vi "Move to New Position.vi"(7 "Curr Filter":i32, 8 "error in (no error)":errorcluster, 9 "Target Filter":i32, 10 "Filter Wheel (0:n-1)":i32, 11 "FW Arduino Control in":refnum<class "FW Arduino Control.lvclass">) -> (0 "error out":errorcluster, 1 "Actual Distance":i32[](array[numeric]), 2 "Log":string, 3 "FW Arduino Control out":refnum<class "FW Arduino Control.lvclass">)   [LabVIEW 2024, in "FW Arduino Control.lvclass"]
uses:
  FW Arduino Control.lvclass
  Filter Wheel Object/Filter Wheel.lvclass
  FW Arduino Control.lvclass/FW Arduino Control.ctl
  <vilib>/Utility/error.llb/Trim Whitespace One-Sided.vi
panel:
  out "notches":i32
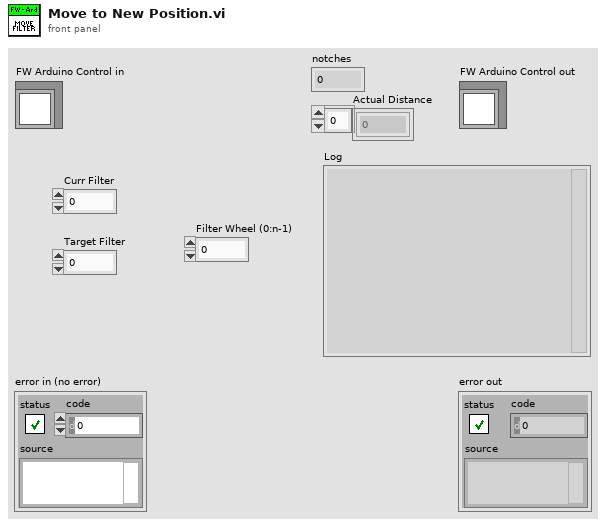
[diagram p1: front panel]
types:
  T1 = typedef "Filter Wheel.lvclass/Filter Wheel configuration.ctl" = cluster{"Num Wheels":i32, "Filters":T2[], "Invalid Combinations":i32[][], "Addr":refnum<visa-resource-name>, "Name":string, "Simulate":bool, "Default Speed":u16, "Homing":T3[]}
  T2 = typedef "Filter Wheel.lvclass/Filter Wheel Details.ctl" = cluster{"Names":string[], "Relative Position":i32[], "Wheel Name":string, "Size":i32}
  T3 = typedef "Filter Wheel Arduino Homing cluster.ctl" = cluster{"Direction (F: CW)":bool, "Speed":i32, "Accel":i32, "Error Cnts":i32, "Homing Delta":i32}
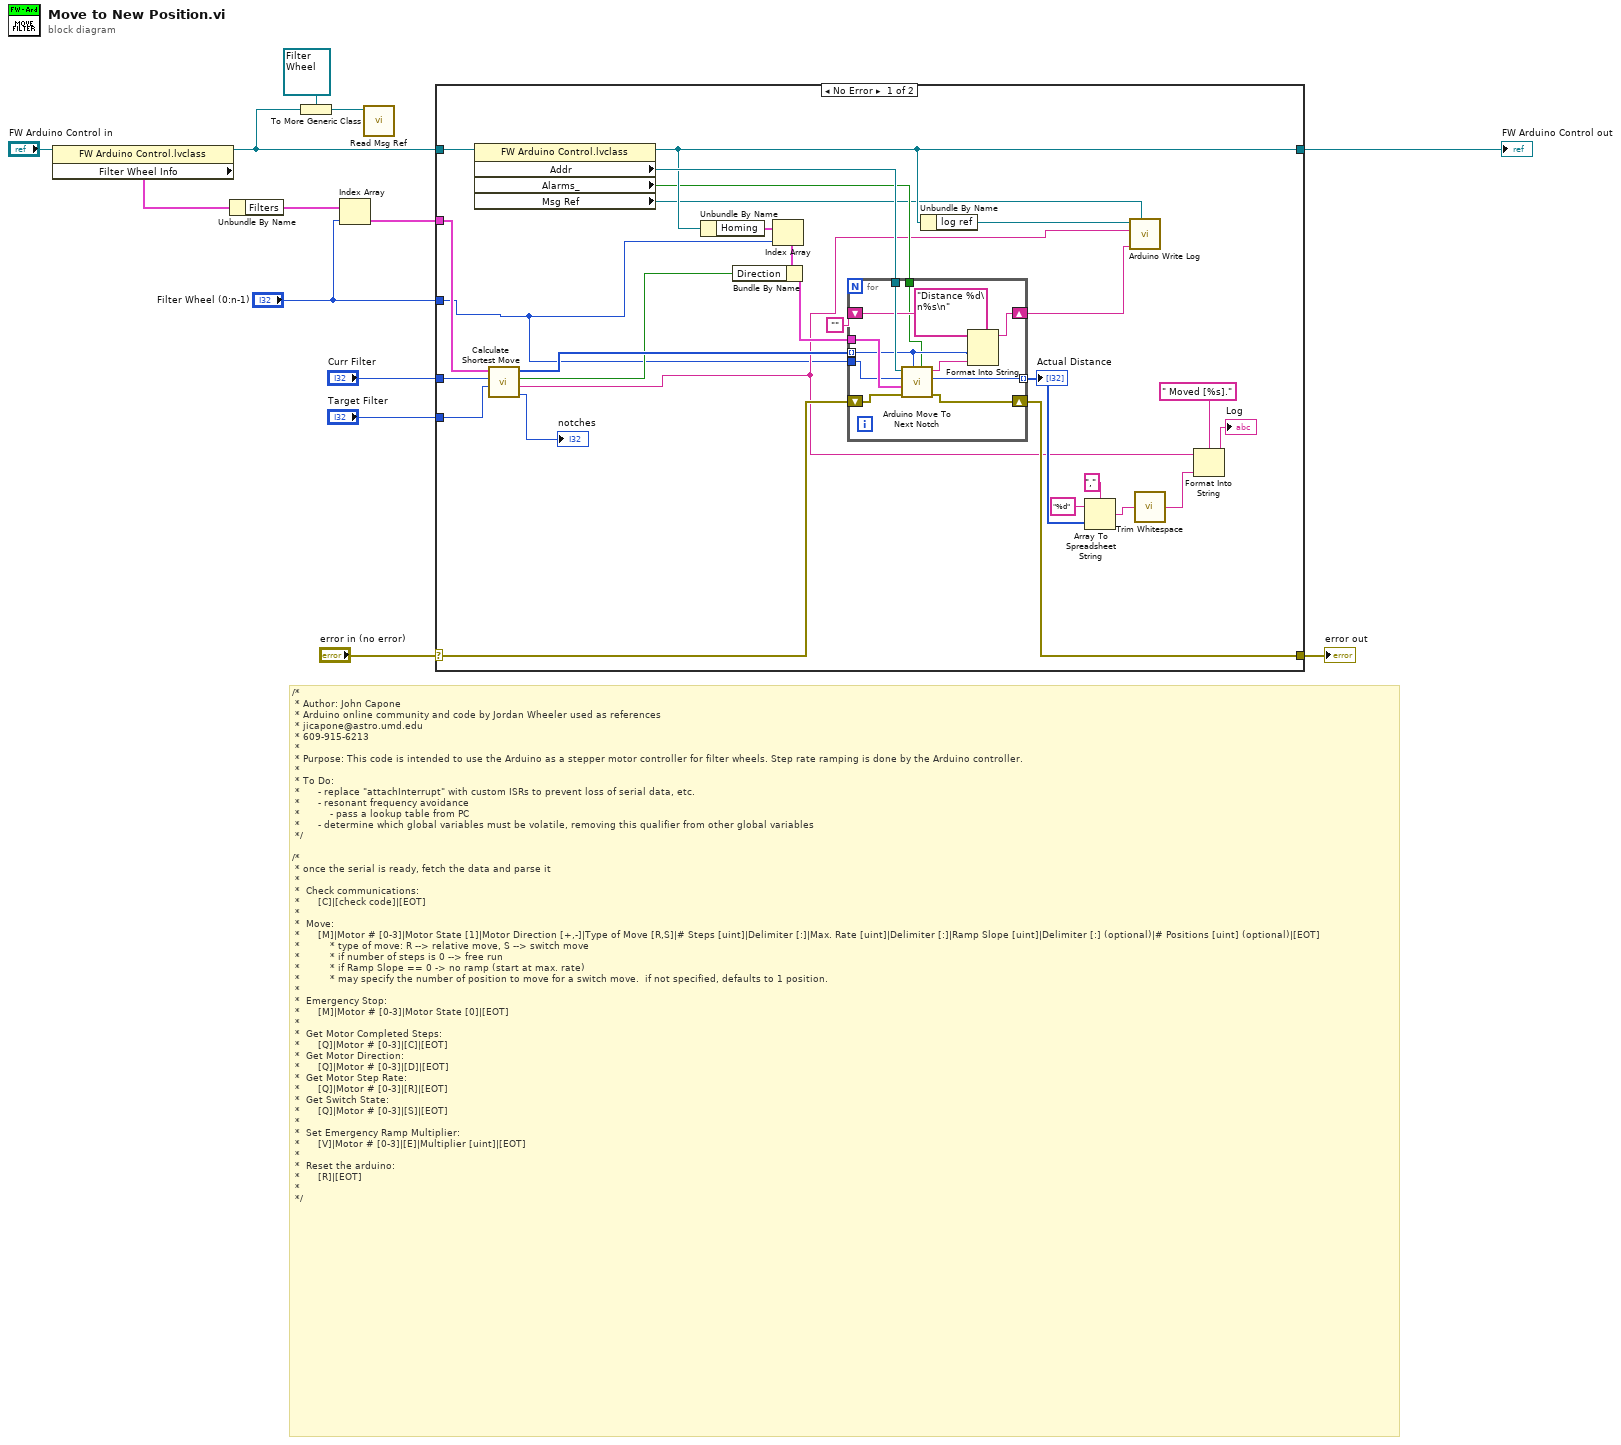
[diagram p0: block diagram]
diagram:
  # "/*\n * Author: John Capone\n * Arduino online community and code by Jordan Wheeler used as references\n * jicapone@astro.umd.edu\n * 609-915-6213\n * \n * Purpose: This code is intended to use the Arduino as a stepper motor controller for filter wheels. Step rate ramping is done by the Arduino controller.\n * \n * To Do:\n *      - replace \"attachInterrupt\" with custom ISRs to prevent loss of serial data, etc.\n *      - resonant frequency avoidance\n *          - pass a lookup table from PC\n *      - determine which global variables must be volatile, removing this qualifier from other global variables\n */\n\n/* \n * once the serial is ready, fetch the data and parse it\n *\n *  Check communications:\n *      [C]|[check code]|[EOT]\n *\n *  Move:\n *      [M]|Motor # [0-3]|Motor State [1]|Motor Direction [+,-]|Type of Move [R,S]|# Steps [uint]|Delimiter [:]|Max. Rate [uint]|Delimiter [:]|Ramp Slope [uint]|Delimiter [:] (optional)|# Positions [uint] (optional)|[EOT]\n *          * type of move: R --> relative move, S --> switch move\n *          * if number of steps is 0 --> free run\n *          * if Ramp Slope == 0 -> no ramp (start at max. rate)\n *          * may specify the number of position to move for a switch move.  if not specified, defaults to 1 position.\n *\n *  Emergency Stop:\n *      [M]|Motor # [0-3]|Motor State [0]|[EOT]\n *\n *  Get Motor Completed Steps:\n *      [Q]|Motor # [0-3]|[C]|[EOT]\n *  Get Motor Direction:\n *      [Q]|Motor # [0-3]|[D]|[EOT]\n *  Get Motor Step Rate:\n *      [Q]|Motor # [0-3]|[R]|[EOT]\n *  Get Switch State:\n *      [Q]|Motor # [0-3]|[S]|[EOT]\n *\n *  Set Emergency Ramp Multiplier:\n *      [V]|Motor # [0-3]|[E]|Multiplier [uint]|[EOT]\n *\n *  Reset the arduino:\n *      [R]|[EOT]\n *\n */"
  n1 = property class="FW Arduino Control.lvclass"(reference="FW Arduino Control in") -> (reference out=w1:refnum<class "FW Arduino Control.lvclass">, "Filter Wheel Info"=w7:T1)  [unwired: 1 in, 1 out]
  n2 = Unbundle By Name(w7) -> ("Filters"=w6:T2[])
  n3 = To More Generic Class(target class=refnum<class "Filter Wheel.lvclass"> refnum ("Filter Wheel.lvclass"), reference=w1) -> (generic class reference=w2:refnum<class "Filter Wheel.lvclass">)
  n4 = Index Array(array=w6, index="Filter Wheel (0:n-1)") -> (element=w4:T2)
  n5 = call-dynamic "Read Msg Ref.vi"("Filter Wheel in"=w2) -> ()  [unwired: 8 in, 3 out]
  n6 = case shown="No Error" "error in (no error)" {
    selector: "error in (no error)" -> [w39 w55]
    tunnel: [w37 w55] -> w12
    tunnel: [w36 w54] -> w9
    tunnel: w1 -> [w41 w54]
    tunnel: "Filter Wheel (0:n-1)" -> [w14 _]
    tunnel: "Curr Filter" -> [w24 _]
    tunnel: "Target Filter" -> [w23 _]
    tunnel: w4 -> [w25 _]
    frame No Error {
      n7 = property class="FW Arduino Control.lvclass"(reference=w41) -> (reference out=w36:refnum<class "FW Arduino Control.lvclass">, "Addr"=w40:refnum<visa-resource-name>, "Alarms_"=w31:bool, "Msg Ref"=w16:refnum<vi>)  [unwired: 1 in, 1 out]
      n8 = call "Calculate Shortest Move.vi"("Target Filter"=w23, "Curr Filter"=w24, "Wheel info"=w25) -> ("notches"=→"notches":i32, "Msg"=w19:string, "direction"=w17:bool, "Moves"=w22:i32[])  [unwired: 5 in]
      n9 = Unbundle By Name(w36) -> ("Homing"=w38:T3[])
      n10 = Index Array(array=w38, index=w14) -> (element=w15:T3)
      n11 = Bundle By Name(cluster=w15, "Direction"=w17) -> (w32:T3)
      n12 = for {
        tunnel: w40 -> [w53]
        tunnel: w32 -> [w52]
        tunnel: w14 -> [w51]
        shift-right: [w49] -> w37
        shift-left: w39 -> [w50]
        shift-right: [w47] -> w34
        shift-left: "" -> [w46]
        tunnel: w22 -> [w44] mode=indexing
        tunnel: w31 -> [w43]
        tunnel: [w42] -> w30 mode=indexing
        n13 = call "Arduino Move To Next Notch.vi"("Ignore Alarm"=w43, "Distance"=w44, "error in"=w50, "Homing Parameters"=w52, "Motor"=w51, "Addr"=w53) -> ("error out"=w49:errorcluster, "Actual distance"=w42:i32, "Log"=w45:string)  [unwired: 3 in]
        n14 = Format Into String(format string="Distance %d\n%s\n", initial string=w46, w44, w45) -> (resulting string=w47:string)  [unwired: 1 in, 1 out]
      }
      "Actual Distance" <- w30
      n15 = Unbundle By Name(w36) -> ("log ref"=w35:refnum<file>)
      n16 = Array To Spreadsheet String(delimiter (Tab)=",", array=w30, 3:"%d" ("format string")) -> (spreadsheet string=w21:string)
      n17 = call "Arduino Write Log.vi"("Msg Ref"=w16, "Arduino data"=w34, "Message"=w19, "log ref"=w35) -> ()  [unwired: 8 in]
      n18 = call <vilib>:"Trim Whitespace.vi"("string"=w21) -> ("trimmed string"=w20:string)  [unwired: 1 in]
      n19 = Format Into String(format string=" Moved [%s].", initial string=w19, w20) -> (resulting string=→"Log":string)  [unwired: 1 in, 1 out]
    }
    frame Error {
    }
  }
  "error out" <- w12
  "FW Arduino Control out" <- w9
